vi "Init(Update ref).vi"(8 "error in (no error)":errorcluster, 11 "Domino Laser module Class in":refnum<class "Domino Laser module Class.lvclass">) -> (0 "error out":errorcluster, 3 "Domino Laser module Class out":refnum<class "Domino Laser module Class.lvclass">)   [LabVIEW 2015, in "Domino LM.lvlib" / "Domino Laser module Class.lvclass"]
uses:
  CTRLS/Domino Laser module Class.lvclass
  CTRLS/Domino Laser module Class.lvclass/Domino Laser module Class.ctl
  ORG_SRL_CTRL/GLB_VAR.vi
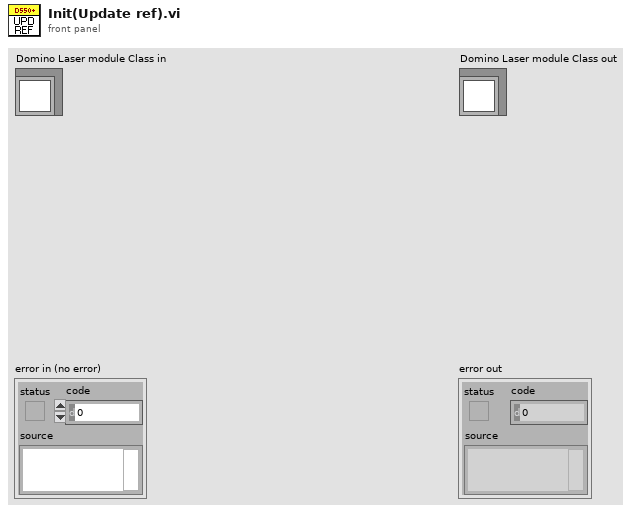
[diagram p1: front panel]
types:
  T1 = cluster{"User":cluster{"Username":refnum<vi>, "Password":refnum<vi>, "Current user":refnum<vi>, "user level":refnum<vi>, "Error MSG":refnum<vi>}, "Main":cluster{"Main Image":refnum<vi>, "Final Carton Status":refnum<vi>, "DM Status":refnum<vi>, "Serial Status":refnum<vi>, "Reject Reason":refnum<vi>, "Total Results":refnum<vi>, "Last Start Results":refnum<vi>, "DM Contents":refnum<vi>, "Motor Speed":refnum<vi>, "Batch Data":refnum<vi>, "Motor Status":refnum<vi>, "Stop Batch":refnum<vi>, "Start Batch":refnum<vi>, "Tab Control":refnum<vi>, "Check USB License":refnum<vi>, "OCV Status":refnum<vi>}, "Recipe":cluster{"Recipe_Carton":refnum<vi>, "Recipe_Printer":refnum<vi>, "Recipe_camera":refnum<vi>, "Carton Config":refnum<vi>, "Layout Config":refnum<vi>, "DM Elements":refnum<vi>, "IMG Config":refnum<vi>, "carton apply sucess":refnum<vi>, "Printer apply sucess":refnum<vi>, "Camera apply sucess":refnum<vi>, "DM Grade":refnum<vi>, "Line Elements":refnum<vi>, "Recipe Configuration":refnum<vi>, "Recipe Data":refnum<vi>, "Idle Button Enable":refnum<vi>, "OCV Selection":refnum<vi>}, "Debug":cluster{"RT setpoints sucess":refnum<vi>, "speed mapping success ":refnum<vi>, "DM Search Options":refnum<vi>, "Speed Mapping":refnum<vi>, "Alarm Override":refnum<vi>, "Main Conv Speed":refnum<vi>, "PLC Settings":refnum<vi>, "Controller Setpoints":refnum<vi>, "Gate Location":refnum<vi>, "Image  Counter":refnum<vi>, "Signature  Counter":refnum<vi>, "Carton Width PLC [MM]":refnum<vi>, "Controller Inputs":refnum<vi>, "Controller Outputs":refnum<vi>}, "System":cluster{"Printer":refnum<vi>, "Printer apply sucess":refnum<vi>, "Camera apply sucess":refnum<vi>, "RT apply sucess":refnum<vi>, "Printer system sucess":refnum<vi>, "Camera Settings":refnum<vi>, "Camera system apply btn":refnum<vi>, "live img":refnum<vi>, "Scanner Settings":refnum<vi>, "Scanner apply sucess":refnum<vi>, "Scanner A Last MSG":refnum<vi>, "Scanner B Last MSG":refnum<vi>, "Emergency":refnum<vi>, "Shrould":refnum<vi>, "Printer Status":refnum<vi>}, "Audit trail":cluster{"Audit filter cluster":refnum<vi>, "Audit Table":refnum<vi>}, "Batch":cluster{"New Workorder Data":refnum<vi>, "Edit Batch":refnum<vi>, "Close Batch":refnum<vi>, "Open Batch":refnum<vi>, "Create Batch":refnum<vi>, "SSCC Config":refnum<vi>}}
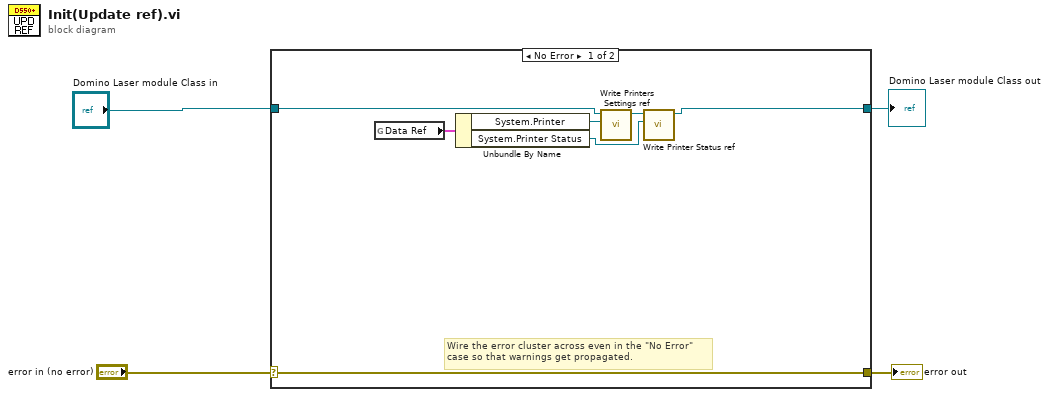
[diagram p0: block diagram]
diagram:
  n1 = case shown="No Error" "error in (no error)" {
    selector: "error in (no error)" -> [w11 w13]
    tunnel: [w11 w13] -> w3
    tunnel: [w6 w12] -> w1
    tunnel: "Domino Laser module Class in" -> [w9 w12]
    frame No Error {
      # "Wire the error cluster across even in the \"No Error\"\ncase so that warnings get propagated."
      n2 = global read "GLB_VAR.vi" "Data Ref"() -> (w10:T1)
      n3 = Unbundle By Name(w10) -> ("System.Printer"=w7:refnum<vi>, "System.Printer Status"=w5:refnum<vi>)
      n4 = call "Write Printers Settings ref.vi"("Printers Settings ref"=w7, "Domino Laser module Class in"=w9) -> ("Domino Laser module Class out"=w8:refnum<class "Domino Laser module Class.lvclass">)  [unwired: 8 in, 1 out]
      n5 = call "Write Printer Status ref.vi"("Printer Status ref"=w5, "Domino Laser module Class in"=w8) -> ("Domino Laser module Class out"=w6:refnum<class "Domino Laser module Class.lvclass">)  [unwired: 8 in, 1 out]
    }
    frame Error {
    }
  }
  "error out" <- w3
  "Domino Laser module Class out" <- w1
